vi "Get Dictionary.vi"(8 "error in (no error)":errorcluster, 11 "Store in":refnum<class "Store.lvclass">) -> (0 "error out":errorcluster, 2 "Dictionary.lvclass":refnum<class "Dictionary.lvclass">, 3 "Store out":refnum<class "Store.lvclass">)   [LabVIEW 2018, in "Application.lvlib" / "Store.lvclass"]
uses:
  Store.lvclass
  Dictionary Class/Dictionary.lvclass
  Store.lvclass/Store.ctl
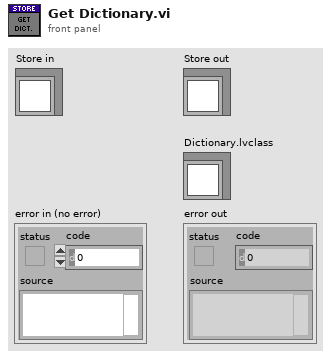
[diagram p1: front panel]
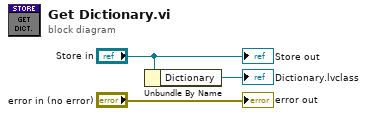
[diagram p0: block diagram]
diagram:
  n1 = Unbundle By Name("Store in") -> ("Dictionary"=→"Dictionary.lvclass":refnum<class "Dictionary.lvclass">)
  "error out" <- "error in (no error)"
  "Store out" <- "Store in"
